vi "Create Message Transport.vi"(7 "Transport Name":string, 8 "error in":errorcluster, 10 "Transport Payload type":refnum<class "IMessagePayload.lvclass">, 11 "NotifierMessageTransport in":refnum<class "NotifierMessageTransport.lvclass">) -> (0 "error out":errorcluster, 3 "NotifierMessageTransport out":refnum<class "NotifierMessageTransport.lvclass">)   [LabVIEW 2016, in "NotifierMessageTransport.lvclass"]
uses:
  NotifierMessageTransport.lvclass
  IMessagePayload/IMessagePayload.lvclass
panel:
  # "INPUTS"
  # "OUTPUTS"
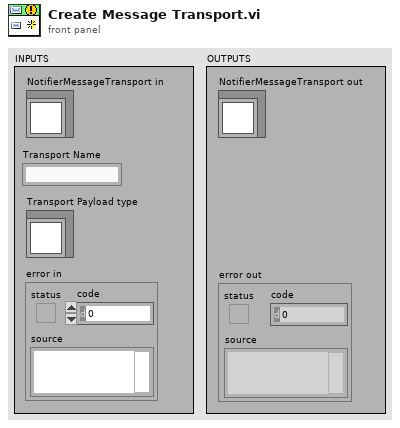
[diagram p1: front panel]
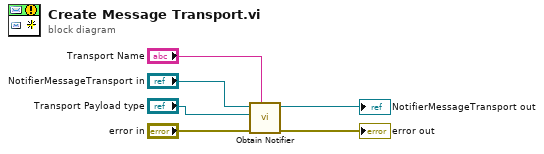
[diagram p0: block diagram]
diagram:
  n1 = call "Obtain Notifier.vi"("Notifier Name"="Transport Name", "error in"="error in", "IMessagePayload.lvclass"="Transport Payload type", "NotifierMessageTransport in"="NotifierMessageTransport in") -> ("error out"=→"error out":errorcluster, "NotifierMessageTransport out"=→"NotifierMessageTransport out":refnum<class "NotifierMessageTransport.lvclass">)  [unwired: 6 in]
